vi "projector_image_to_camera_image.vi"(8 "error in (no error)":errorcluster, 11 "Experiment Folder in":string) -> (0 "error out":errorcluster, 3 "Experiment Folder out":string="C:\\Data\\20200122_launched_from_main_test\\Data20200122_131836")   [LabVIEW 2019]
uses:
  radiucenter2topleftwidthheight.vi
  affine_transform_point.vi
  DebugGlobal.vi
  <vilib>/vision/NI_Vision_Development_Module.lvlib
panel:
  out "processors used":i32
  out "Processing Rate (images / s)":dbl
  out "Display Array":i32[](array[numeric])
  out "Progress %":i32(slide) scale=0.0..100.0
  out "zip elapsed time (s)":i32
  out "conversion elapsed time (s)":i32
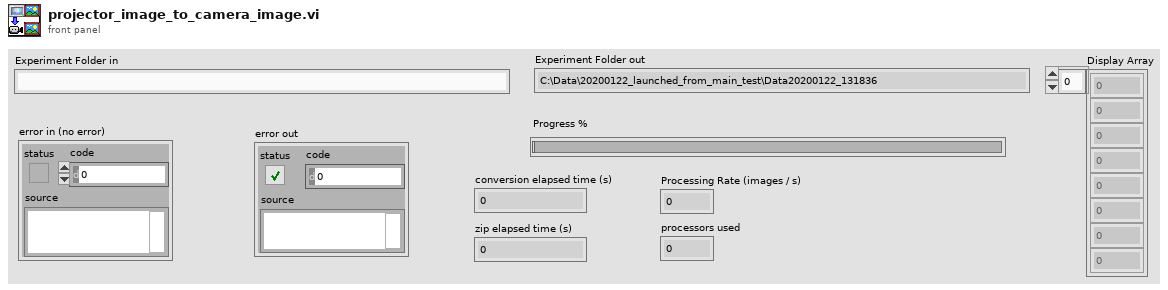
[diagram p1: front panel]
types:
  T1 = typedef "IMAQ Image.ctl" = refnum<image>
  T2 = typedef "Image Type" = u32
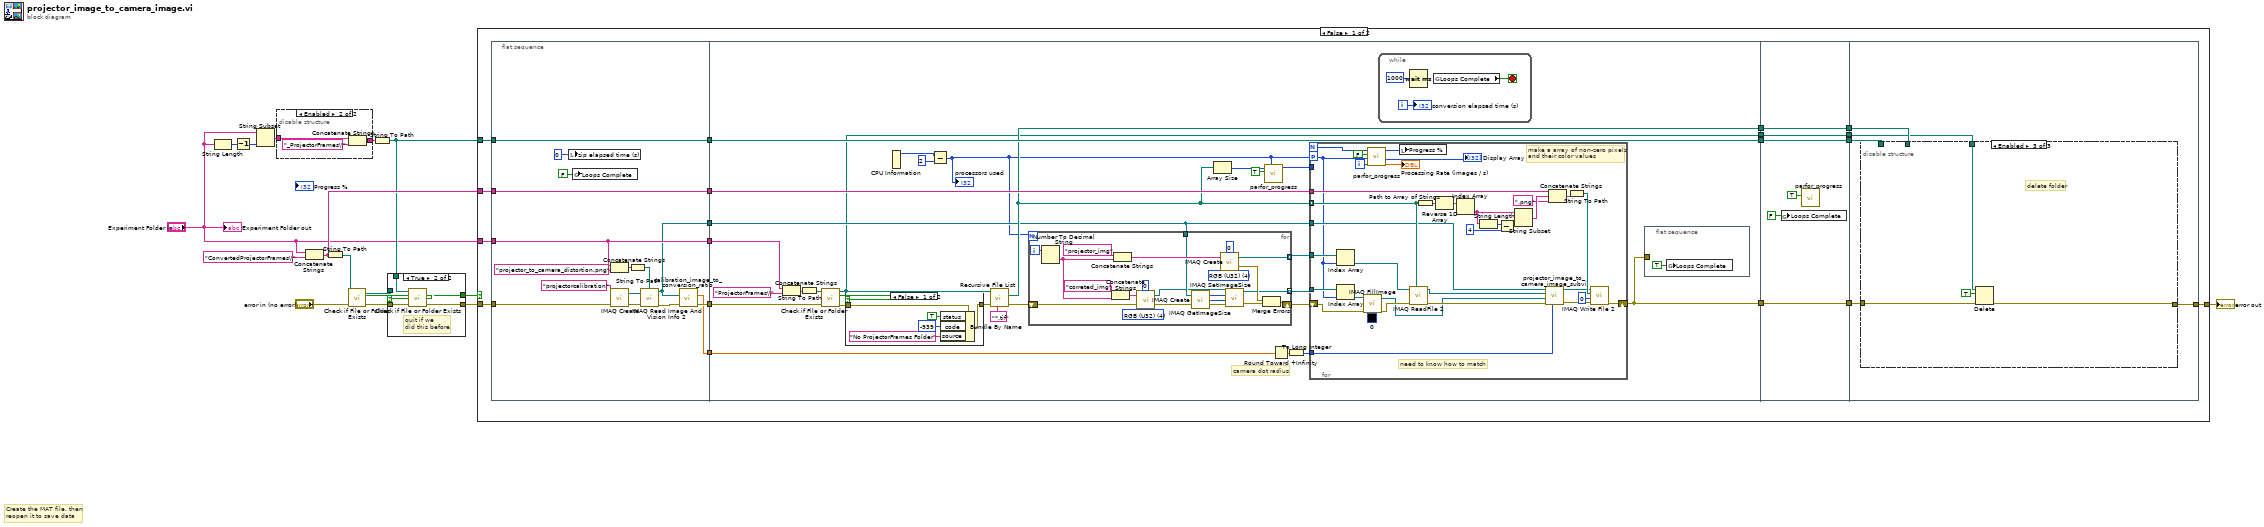
[diagram p0: block diagram]
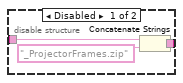
[diagram p2: hidden frame]
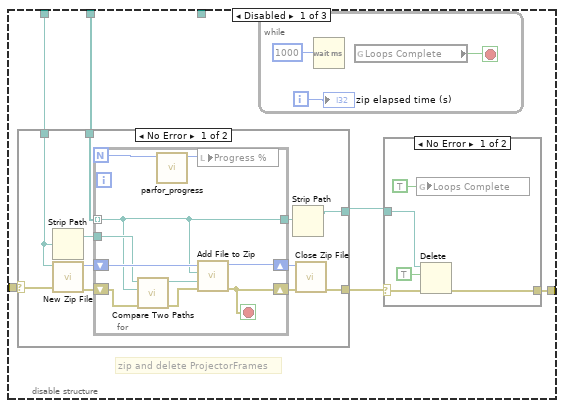
[diagram p4: hidden frame]
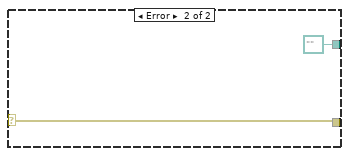
[diagram p5: hidden frame]
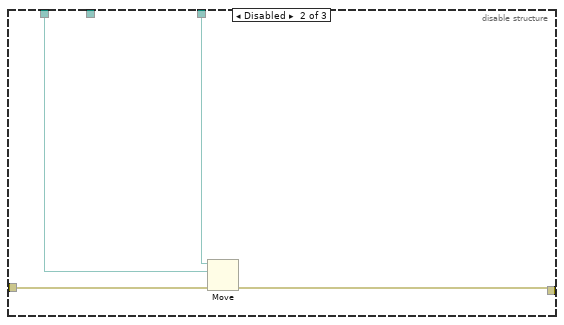
[diagram p7: hidden frame]
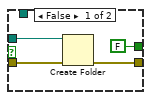
[diagram p9: hidden frame]
diagram:
  # "Create the MAT file, then\nreopen it to save data"
  n1 = String Length(string="Experiment Folder in") -> (length=w8:i32)
  n2 = Decrement(x=w8) -> (x-1=w7:i32)
  n3 = String Subset(string="Experiment Folder in", length (rest)=w7) -> (substring=w6:string)  [unwired: 1 in]
  n4 = disable-structure shown="Enabled" {
    disable-tunnel: w6 -> [w18 w21]
    disable-tunnel: [w17 w22] -> w5
    frame Disabled {
      n5 = Concatenate Strings(w18, "_ProjectorFrames.zip" ("string")) -> (w17:string)
    }
    frame Enabled {
      n6 = Concatenate Strings(w21, "_ProjectorFrames\\" ("string")) -> (w22:string)
    }
  }
  n7 = Concatenate Strings("Experiment Folder in", "ConvertedProjectorFrames\\" ("string")) -> (w10:string)
  n8 = String To Path(string=w10) -> (path=w15:path)
  n9 = call <vilib>:"Check if File or Folder Exists.vi"("error in (no error)"="error in (no error)", "path"=w15) -> ("error out"=w12:errorcluster, "file or folder exists?"=w13:bool, "dup path"=w14:path)  [unwired: 7 in]
  n10 = String To Path(string=w5) -> (path=w4:path)
  n11 = case shown="True" w13 {
    tunnel: w14 -> [w26 _]
    tunnel: [w25 w29] -> w2
    tunnel: w12 -> [w24 w30]
    tunnel: w4 -> [_ w28]
    tunnel: [FALSE ("file or folder exists?") w27] -> w9
    frame False {
      n12 = Create Folder(path (use dialog)=w26, error in=w24) -> (error out=w25:errorcluster)  [unwired: 1 in, 2 out]
    }
    frame True {
      # "quit if we \ndid this before"
      n13 = call <vilib>:"Check if File or Folder Exists.vi"("error in (no error)"=w30, "path"=w28) -> ("error out"=w29:errorcluster, "file or folder exists?"=w27:bool)  [unwired: 7 in, 1 out]
    }
  }
  n14 = case shown="False" w9 {
    tunnel: [w39 w217] -> w16
    tunnel: w2 -> [w38 w217]
    tunnel: "Experiment Folder in" -> [w37 _]
    tunnel: w4 -> [w36 _]
    tunnel: w10 -> [w35 _]
    frame False {
      n15 = flat-sequence {
        tunnel: w37 -> [w55]
        tunnel: w38 -> [w59]
        tunnel: [w52] -> w48
        tunnel: [w55] -> w49
        tunnel: w36 -> [w63]
        tunnel: [w63] -> w47
        tunnel: [w62] -> w46
        tunnel: w35 -> [w62]
        tunnel: [w51] -> w34
        tunnel: [w50] -> w33
        tunnel: [w70] -> w45
        tunnel: [w75] -> w44
        tunnel: [w79] -> w43
        tunnel: w49 -> [w81]
        tunnel: w48 -> [w80]
        tunnel: w47 -> [w79]
        tunnel: w46 -> [w78]
        tunnel: w34 -> [w73]
        tunnel: w33 -> [w72]
        tunnel: [w66] -> w31
        tunnel: w45 -> [w161]
        tunnel: [w161] -> w40
        tunnel: w44 -> [w165]
        tunnel: [w165] -> w41
        tunnel: w43 -> [w164]
        tunnel: [w164] -> w42
        tunnel: [w160] -> w32
        tunnel: w31 -> [w160]
        tunnel: [w170] -> w39
        tunnel: w42 -> [w167]
        tunnel: w41 -> [w168]
        tunnel: w40 -> [w169]
        tunnel: w32 -> [w166]
        frame #0 {
          n16 = local write "zip elapsed time (s)"(0 ("zip elapsed time (s)")) -> ()
          n17 = global write "DebugGlobal.vi" "Loops Complete"(FALSE ("Loops Complete")) -> ()
          n18 = Concatenate Strings(w55, "projector_to_camera_distortion.png" ("string")) -> (w56:string)
          n19 = call "IMAQ Create"("Image Name"="projectorcalibration", "error in (no error)"=w59) -> ("New Image"=w58:T1, "error out"=w61:errorcluster)  [unwired: 3 in]
          n20 = String To Path(string=w56) -> (path=w54:path)
          n21 = call "IMAQ Read Image And Vision Info 2"("File Path"=w54, "error in (no error)"=w61, "Image"=w58) -> ("error out"=w53:errorcluster, "Image Out"=w51:T1)  [unwired: 6 in, 1 out]
          n22 = call "calibration_image_to_conversion_ratio.vi"("error in (no error)"=w53, "Calibration Image"=w51) -> ("error out"=w52:errorcluster, "conversion ratio"=w50:dbl)  [unwired: 8 in]
        }
        frame #1 {
          # "camera dot radius"
          n23 = Concatenate Strings(w81, "ProjectorFrames\\" ("string")) -> (w86:string)
          n24 = String To Path(string=w86) -> (path=w85:path)
          n25 = call <vilib>:"Check if File or Folder Exists.vi"("error in (no error)"=w80, "path"=w85) -> ("error out"=w83:errorcluster, "file or folder exists?"=w84:bool, "dup path"=w66:path)  [unwired: 7 in]
          n26 = case shown="False" w84 {
            tunnel: w83 -> [w136 w137]
            tunnel: [w132 w137] -> w82
            frame False {
              n27 = Bundle By Name(cluster=w136, "status"=TRUE, "code"=-939, "source"="No ProjectorFrames Folder") -> (w132:errorcluster)
            }
            frame True {
            }
          }
          n28 = CPU Information() -> (4:w69:i32)  [unwired: 3 out]
          n29 = Subtract(x=w69, y=2) -> (x-y=w67:i32)
          "processors used" <- w67
          n30 = call <vilib>:"Recursive File List.vi"("pattern"="*.tif", "error in (no error)"=w82, "Folder Path"=w66) -> ("error out"=w92:errorcluster, "All Files in Dir"=w75:path[])  [unwired: 4 in, 3 out]
          n31 = for {
            N: w67 -> [_]
            shift-right: [w156] -> w71
            shift-left: w92 -> [w138]
            tunnel: [w155] -> w90 mode=indexing
            tunnel: [w139] -> w91 mode=indexing
            tunnel: w73 -> [w143]
            i -> [w157]
            w147 = T2 4 items=["Grayscale (U8)", "Grayscale (I16)", "Grayscale (SGL)", "Complex (CSG)", "RGB (U32)", "HSL (U32)", "RGB (U64)", "Grayscale (U16)"] ("Image Type")
            w148 = T2 4 items=["Grayscale (U8)", "Grayscale (I16)", "Grayscale (SGL)", "Complex (CSG)", "RGB (U32)", "HSL (U32)", "RGB (U64)", "Grayscale (U16)"] ("Image Type")
            n32 = Number To Decimal String(number=w157) -> (decimal integer string=w152:string)  [unwired: 1 in]
            n33 = Concatenate Strings("correted_img", w152) -> (w154:string)
            n34 = Concatenate Strings("projector_img", w152) -> (w158:string)
            n35 = call "IMAQ Create"("Border Size"=0, "Image Name"=w154, "Image Type"=w147, "error in (no error)"=w138) -> ("New Image"=w140:T1, "error out"=w142:errorcluster)  [unwired: 1 in]
            n36 = call "IMAQ GetImageSize"("Image"=w143, "error in (no error)"=w142) -> ("Y Resolution"=w144:i32, "X Resolution"=w145:i32, "error out"=w146:errorcluster)  [unwired: 2 in]
            n37 = call "IMAQ Create"("Border Size"=0, "Image Name"=w158, "Image Type"=w148) -> ("New Image"=w155:T1, "error out"=w151:errorcluster)  [unwired: 2 in]
            n38 = call "IMAQ SetImageSize"("error in (no error)"=w146, "Y Resolution"=w144, "X Resolution"=w145, "Image"=w140) -> ("error out"=w141:errorcluster, "Image Out"=w139:T1)  [unwired: 1 in]
            n39 = Merge Errors(w151, w141) -> (w156:errorcluster)
          }
          n40 = Array Size(array=w75) -> (size(s)=w74:i32)
          n41 = call "parfor_progress.vi"("Parpool Count"=w67, "reset"=TRUE, "N"=w74) -> ("Percent Count"=w76:i32)  [unwired: 6 in, 2 out]
          n42 = Round Toward +Infinity(x=w72) -> ()  [unwired: 1 out]
          n43 = To Long Integer(number=w72) -> (32bit integer=w89:i32)
          n44 = for {
            N -> [w120]
            tunnel: w75 -> [w131] mode=indexing
            tunnel: w90 -> [w128]
            tunnel: w73 -> [w130]
            tunnel: w91 -> [w129]
            tunnel: w89 -> [w108]
            workers-P: w67 -> [w115]
            tunnel: w78 -> [w118]
            tunnel: w76 -> [_]
            shift-right: [w109] -> w70
            shift-left: w71 -> [w105]
            i -> [w116]
            # "need to know how to match"
            # "make a array of non-zero pixels\nand their color values"
            n45 = Index Array(array=w128, index=w115) -> (element=w127:T1)
            n46 = Index Array(array=w129, index=w115) -> (element=w106:T1)
            n47 = call "IMAQ FillImage"("Color Pixel Value"=u32 0, "error in (no error)"=w105, "Image"=w106) -> ("error out"=w104:errorcluster, "Image Out"=w103:T1)  [unwired: 7 in]
            n48 = call "parfor_progress.vi"("Current Display"=w116, "PID"=w115, "reset"=FALSE, "N"=w120) -> ("Processing Rate"=→"Processing Rate (images / s)":dbl, "Display Array"=→"Display Array":i32[], "Percent Count"=w119:i32)  [unwired: 5 in]
            n49 = local write "Progress %"(w119) -> ()
            n50 = call "IMAQ ReadFile 2"("File Path"=w131, "error in (no error)"=w104, "Image"=w127) -> ("error out"=w124:errorcluster, "Image Out"=w112:T1)  [unwired: 4 in, 3 out]
            n51 = Path to Array of Strings(0:w131) -> (2:w123:string[])  [unwired: 1 out]
            n52 = Reverse 1D Array(array=w123) -> (reversed array=w122:string[])
            n53 = Index Array(array=w122) -> (element=w102:string)  [unwired: 1 in]
            n54 = String Length(string=w102) -> (length=w101:i32)
            n55 = Subtract(x=w101, y=4) -> (x-y=w100:i32)
            n56 = String Subset(string=w102, length (rest)=w100) -> (substring=w98:string)  [unwired: 1 in]
            n57 = call "projector_image_to_camera_image_subvi.vi"("Camera dot radius"=w108, "error in (no error)"=w124, "Converted Camera Image In"=w103, "Projector Image In"=w112, "Projector to Camera Calibration"=w130) -> ("error out"=w111:errorcluster, "Converted Camera Image Out"=w110:T1)  [unwired: 5 in]
            n58 = Concatenate Strings(w118, w98, ".png" ("string")) -> (w121:string)
            n59 = String To Path(string=w121) -> (path=w126:path)
            n60 = call-poly "IMAQ Write File 2"("error in (no error)"=w111, "Image Quality"=u32 0, "File Path"=w126, "Image"=w110) -> ("error out"=w109:errorcluster)  [unwired: 6 in, 1 out]
          }
          n61 = while {
            i -> [w95]
            stop <- w94 stop-if-true
            n62 = Wait (ms)(milliseconds to wait=u32 1000 ("y")) -> ()  [unwired: 1 out]
            n63 = global read "DebugGlobal.vi" "Loops Complete"() -> (w94:bool)
            "conversion elapsed time (s)" <- w95
          }
          n64 = flat-sequence {
            tunnel: w70 -> [_]
            frame #0 {
              n65 = global write "DebugGlobal.vi" "Loops Complete"(TRUE ("Loops Complete")) -> ()
            }
          }
        }
        frame #2 {
          n66 = global write "DebugGlobal.vi" "Loops Complete"(FALSE ("Loops Complete")) -> ()
          n67 = call "parfor_progress.vi"("reset"=TRUE) -> ()  [unwired: 8 in, 3 out]
        }
        frame #3 {
          n68 = disable-structure shown="Enabled" {
            disable-tunnel: [w176 w209 w214] -> w170
            disable-tunnel: w169 -> [w175 w212 w216]
            disable-tunnel: w168 -> [w172 _ _]
            disable-tunnel: w167 -> [w171 w211 _]
            disable-tunnel: w166 -> [_ w210 w215]
            frame Disabled {
              # "zip and delete ProjectorFrames"
              n69 = case shown="No Error" w175 {
                selector: w175 -> [w187 w202]
                tunnel: [w185 w202] -> w174
                tunnel: [w183 path "" ("stripped path")] -> w173
                tunnel: w171 -> [w181 _]
                tunnel: w172 -> [w180 _]
                frame No Error {
                  n70 = Strip Path(path=w181) -> (stripped path=w188:path)  [unwired: 1 out]
                  n71 = call <vilib>:"New Zip File.vi"("error in (no error)"=w187, "target"=w181) -> ("error out"=w190:errorcluster, "zip file out"=w189:i64)  [unwired: 3 in, 1 out]
                  n72 = for {
                    N -> [w192]
                    tunnel: w180 -> [w193] mode=indexing
                    shift-right: [w199] -> w184
                    shift-left: w189 -> [w200]
                    shift-right: [w196] -> w186
                    shift-left: w190 -> [w198]
                    tunnel: w188 -> [w195]
                    tunnel: [w193] -> w182
                    stop <- w196 stop-if-true
                    n73 = call <vilib>:"Compare Two Paths.vi"("error in (no error)"=w198, "Path 2"=w193, "Path 1"=w195) -> ("error out"=w197:errorcluster, "Relative Path from 1 to 2"=w194:path)  [unwired: 5 in, 2 out]
                    n74 = call "parfor_progress.vi"("N"=w192) -> ("Percent Count"=w191:i32)  [unwired: 8 in, 2 out]
                    n75 = local write "Progress %"(w191) -> ()
                    n76 = call <vilib>:"Add File to Zip.vi"("error in (no error)"=w197, "destination path in zip"=w194, "source file path"=w193, "zip file in"=w200) -> ("error out"=w196:errorcluster, "zip file out"=w199:i64)  [unwired: 6 in]
                  }
                  n77 = Strip Path(path=w182) -> (stripped path=w183:path)  [unwired: 1 out]
                  n78 = call <vilib>:"Close Zip File.vi"("error in (no error)"=w186, "zip file in"=w184) -> ("error out"=w185:errorcluster)  [unwired: 1 in, 4 out]
                }
                frame Error {
                }
              }
              n79 = while {
                i -> [w177]
                stop <- w178 stop-if-true
                n80 = Wait (ms)(milliseconds to wait=u32 1000 ("y")) -> ()  [unwired: 1 out]
                n81 = global read "DebugGlobal.vi" "Loops Complete"() -> (w178:bool)
                "zip elapsed time (s)" <- w177
              }
              n82 = case shown="No Error" w174 {
                selector: w174 -> [w206 w208]
                tunnel: [w205 w208] -> w176
                tunnel: w173 -> [w204 _]
                frame No Error {
                  n83 = global write "DebugGlobal.vi" "Loops Complete"(TRUE ("Loops Complete")) -> ()
                  n84 = Delete(path (use dialog)=w204, entire hierarchy (F)=TRUE, error in=w206) -> (error out=w205:errorcluster)  [unwired: 2 in, 2 out]
                }
                frame Error {
                }
              }
            }
            frame Disabled {
              n85 = Move(source path=w210, error in=w212, 10:w211) -> (error out=w209:errorcluster)  [unwired: 2 in, 2 out]
            }
            frame Enabled {
              # "delete folder"
              n86 = Delete(path (use dialog)=w215, entire hierarchy (F)=TRUE, error in=w216) -> (error out=w214:errorcluster)  [unwired: 2 in, 2 out]
            }
          }
        }
      }
    }
    frame True {
    }
  }
  "error out" <- w16
  "Experiment Folder out" <- "Experiment Folder in"
